vi "Write new location of new page to previous page.vi"(8 "Location in byte stream of the \nnew IFD":u32, 11 "Image Data in":u8[](array[numeric])) -> (2 "Location of the \nlast page's \n\"next IFD pointer\"":i32, 3 "Image Data out":u8[](array[numeric]))   [LabVIEW 2015, in "Tiff reader.lvlib"]
doc: "This .vi changes the last IFD pointer in the input Data array to point to a new IFD location. This is necessary to stitch (merge) TIFF files together into a stack."
uses:
  Tiff reader.lvlib
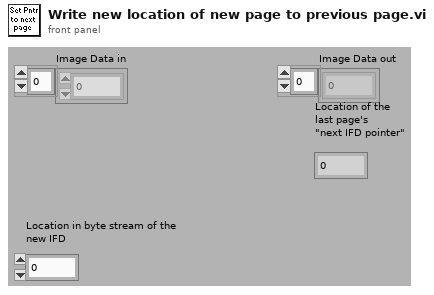
[diagram p1: front panel]
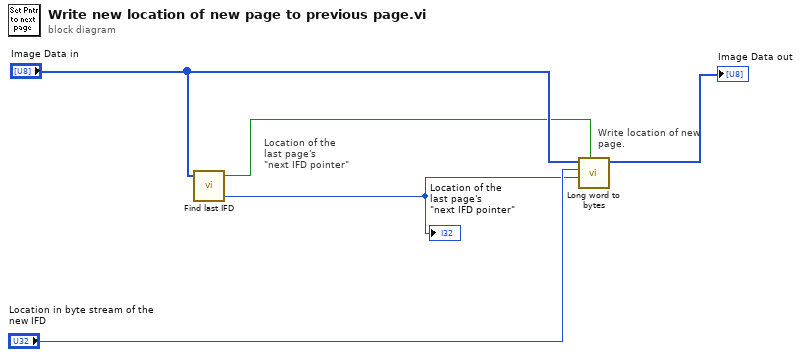
[diagram p0: block diagram]
diagram:
  # "Write location of new\npage."
  # "Location of the \nlast page's \n\"next IFD pointer\""
  n1 = call "Find last IFD.vi"("TIFF Data in"="Image Data in") -> ("Location in byte stream of last IFD pointer.  This\nis the word to change if you are adding another page\nto the file."=w3:i32, "Litt/BigEnd"=w1:bool)  [unwired: 3 out]
  "Location of the \nlast page's \n\"next IFD pointer\"" <- w3
  n2 = call "Long word to bytes.vi"("Litt/BigEnd"=w1, "Index"=w3, "U32"="Location in byte stream of the \nnew IFD", "Image Data in"="Image Data in") -> ("Image Data out"=→"Image Data out":u8[])  [unwired: 5 out]
